vi "RC_test_reader.vi"(8 "error in (no error)":errorcluster, 9 "Motors IDs Found":u8[](array[numeric]), 10 "Read positions (dyn)":dbl[](array[numeric]), 11 "VISA Refnum in":refnum<visa-resource-name>) -> (0 "error out":errorcluster[](array[cluster]), 1 "Motors Read Correctly":bool[](array[boolean]), 2 "Dynamixel Positions (deg)":dbl[](array[numeric]), 3 "Read positions latest (dyn)":dbl[](array[numeric]), 5 "VISA Refnum OUT":refnum<visa-resource-name>)   [LabVIEW 2013]
doc: "This VI takes an array of motor IDs and reads the position of each one. It outputs as both raw values and as degrees.\n\nIt's set up for the SAIL Dynamixels, because it scales by 360/1200. We're still investigating whether the rudder has different units."
uses:
  <instrlib>/Dynamixel Motor/Dynamixel Motor.lvlib
panel:
  in  "Rudder ID":u8
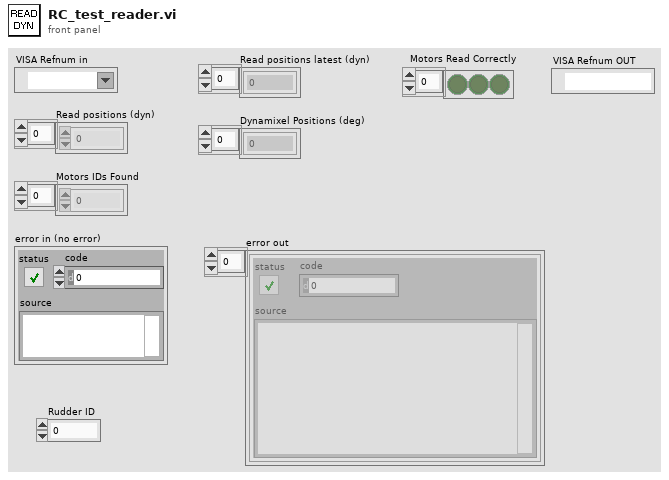
[diagram p1: front panel]
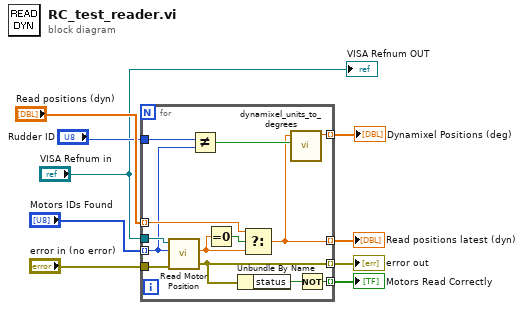
[diagram p0: block diagram]
diagram:
  n1 = for {
    tunnel: "VISA Refnum in" -> [w22]
    tunnel: "Motors IDs Found" -> [w17] mode=indexing
    tunnel: "error in (no error)" -> [w21]
    tunnel: [w12] -> w8 mode=indexing
    tunnel: "Read positions (dyn)" -> [w18] mode=indexing
    tunnel: [w15] -> w5 mode=indexing
    tunnel: [w14] -> w4 mode=indexing
    tunnel: "Rudder ID" -> [w13]
    tunnel: [w10] -> w2 mode=indexing
    n2 = call <instrlib>:"Read Motor Position.vi"("error in (no error)"=w21, "Motor ID (0)"=w17, "VISA resource name"=w22) -> ("error out"=w12:errorcluster, "Position (deg)"=w19:dbl)  [unwired: 6 in, 1 out]
    n3 = Not Equal?(x=w13, y=w17) -> (x != y?=w16:bool)
    n4 = Equal To 0?(x=w19) -> (x = 0?=w20:bool)
    n5 = Unbundle By Name(w12) -> ("status"=w11:bool)
    n6 = Select(t=w18, s=w20, f=w19) -> (s? t:f=w15:dbl)
    n7 = call "dynamixel_units_to_degrees.vi"("MX Motor? (T)"=w16, "Dynamixel Input"=w15) -> ("Degrees"=w14:dbl)  [unwired: 8 in, 1 out]
    n8 = Not(x=w11) -> (.not. x?=w10:bool)
  }
  "Read positions latest (dyn)" <- w5
  "Dynamixel Positions (deg)" <- w4
  "error out" <- w8
  "Motors Read Correctly" <- w2
  "VISA Refnum OUT" <- "VISA Refnum in"
